vi "DAQ.vi"(8 "error in":errorcluster, 11 "Detector in":refnum<class "PID.lvclass">) -> (0 "error out":errorcluster, 2 "data":dbl[](array[numeric]), 3 "Detector out":refnum<class "PID.lvclass">)   [LabVIEW 2011, in "PID.lvclass"]
doc: "Fetch the latest available spectrum."
uses:
  PID.lvclass
  <vilib>/Analysis/NI_AALPro.lvlib
  <vilib>/ptbypt/NI_PtbyPt.lvlib
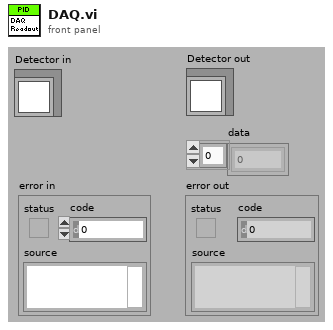
[diagram p1: front panel]
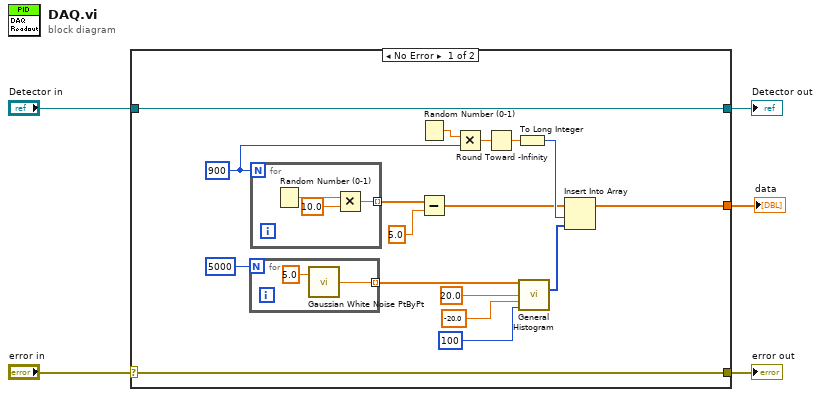
[diagram p0: block diagram]
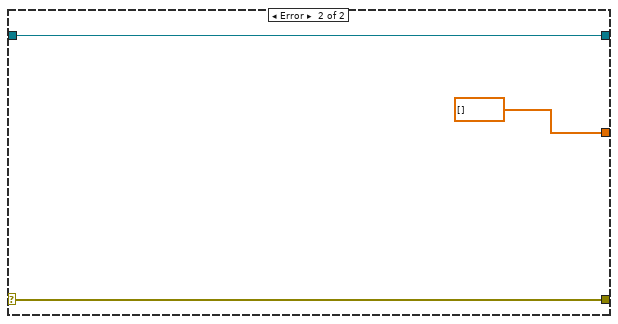
[diagram p2: hidden frame]
diagram:
  n1 = case shown="No Error" "error in" {
    selector: "error in" -> [w21 w30]
    tunnel: [w21 w30] -> w4
    tunnel: [w22 w29] -> w2
    tunnel: "Detector in" -> [w22 w29]
    tunnel: [w6 dbl[] []] -> w1
    frame No Error {
      w9 = 900
      n2 = for {
        N: 5000 -> [_]
        tunnel: [w23] -> w10 mode=indexing
        n3 = call <vilib>:"Gaussian White Noise PtByPt.vi"("standard deviation"=5.0) -> ("Gaussian white noise"=w23:dbl)  [unwired: 2 in]
      }
      n4 = for {
        N: w9 -> [_]
        tunnel: [w25] -> w14 mode=indexing
        n5 = Random Number (0-1)() -> (number: 0 to 1=w27:dbl)
        n6 = Multiply(x=w27, y=10.0) -> (x*y=w25:dbl)
      }
      n7 = Random Number (0-1)() -> (number: 0 to 1=w17:dbl)
      n8 = Subtract(x=w14, y=5.0) -> (x-y=w12:dbl[])
      n9 = Multiply(x=w17, y=w9) -> (x*y=w7:dbl)
      n10 = Round Toward -Infinity(1:w7) -> (0:w8:dbl)
      n11 = To Long Integer(number=w8) -> (32bit integer=w16:i32)
      n12 = call <vilib>:"General Histogram.vi"("X"=w10, "max"=20.0, "min"=-20.0, "# bins"=100) -> ("Histogram"=w15:i32[])  [unwired: 7 in, 4 out]
      n13 = Insert Into Array(array=w12, index=w16, new element=w15) -> (w6:dbl[])
    }
    frame Error {
    }
  }
  "error out" <- w4
  "Detector out" <- w2
  "data" <- w1
